vi "Software triggered acquisition - polling.vi"() -> ()   [LabVIEW 2015]
uses:
  SubVIs/Parameters Get & Set/Set Parameters/Set Gain.vi
  SubVIs/Parameters Get & Set/Get Parameters/Get NumberOfQueuedFrames.vi
  SubVIs/Parameters Get & Set/Set Parameters/Set ExposureTime_us.vi
  SubVIs/Parameters Get & Set/Set Parameters/Set FramesPerTrigger_zeroForUnlimited.vi
  SubVIs/Parameters Get & Set/Set Parameters/Set OperationMode.vi
  C:/code/Host/Installer/Scientific Camera Interfaces/LabVIEW/64_bit/Library_X64/Thorlabs.TSI.TLCameraInterfaces.dll
  64_bit/Library_X64/Thorlabs.TSI.TLCameraInterfaces.dll
panel:
  in  "Exposure (ms)":u32=100
  in  "Gain":u32 max=1023
  in  "Trigger Button":bool
  in  "stop":bool
  out "Intensity Graph Mono":u16[][](graph)
  out "FrameNumber":u32
  in  "Frames Per Trigger":u32=1
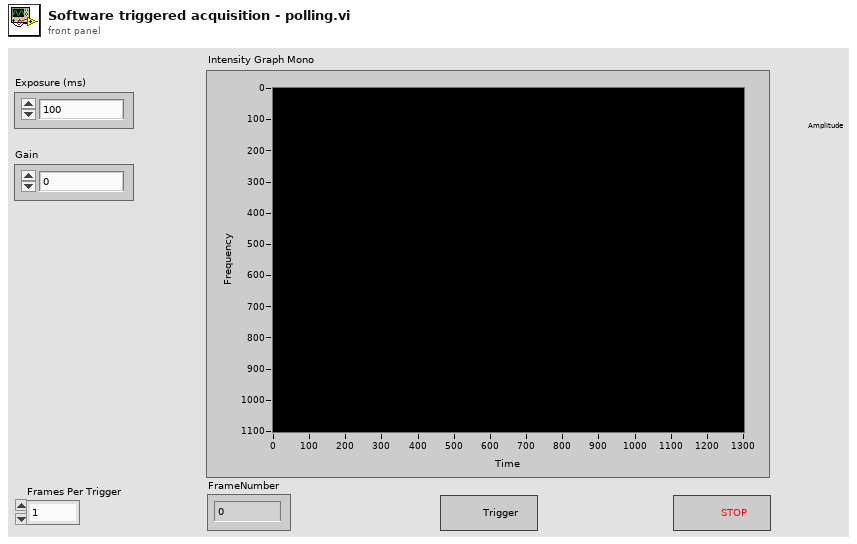
[diagram p1: front panel]
types:
  T1 = enum8{"Enabled", "Disabled", "Disabled and Grayed Out"}
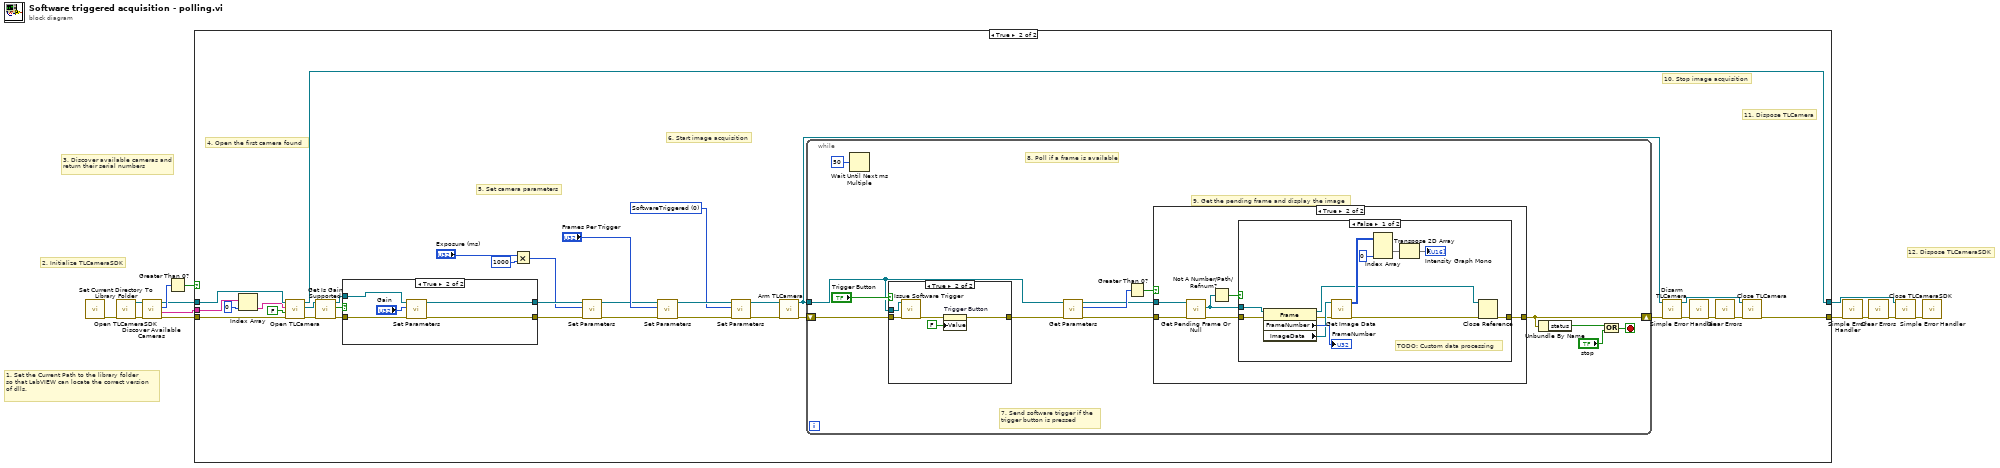
[diagram p0: block diagram]
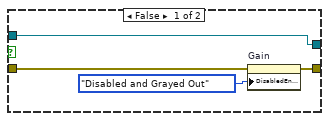
[diagram p3: hidden frame]
diagram:
  # "1. Set the Current Path to the library folder\nso that LabVIEW can locate the correct version\nof dlls."
  # "12. Dispose TLCameraSDK"
  # "3. Discover available cameras and\nreturn their serial numbers"
  # "2. Initialize TLCameraSDK"
  n1 = call "Set Current Directory To Library Folder.vi"() -> ("error out"=w7:errorcluster)  [unwired: 11 in]
  n2 = call "Open TLCameraSDK.vi"("error in (no error)"=w7) -> ("error out"=w6:errorcluster, "Thorlabs.TSI.TLCameraInterfaces.ITLCameraSDK"=w5:refnum<k24>)  [unwired: 9 in]
  n3 = call "Discover Available Cameras.vi"("error in (no error)"=w6, "Thorlabs.TSI.TLCameraInterfaces.ITLCameraSDK"=w5) -> ("error out"=w9:errorcluster, "Serial Numbers"=w11:string[], "Number of Cameras"=w13:i32, "Thorlabs.TSI.TLCameraInterfaces.ITLCameraSDK"=w10:refnum<k24>)  [unwired: 6 in]
  n4 = Greater Than 0?(x=w13) -> (x > 0?=w12:bool)
  n5 = case shown="True" w12 {
    tunnel: w11 -> [_ w48]
    tunnel: w10 -> [w14 w43]
    tunnel: w9 -> [w15 w32]
    tunnel: [w15 w30] -> w2
    tunnel: [w14 w42] -> w8
    frame False {
    }
    frame True {
      w18 = 0 items=["SoftwareTriggered", "HardwareTriggered", "Bulb", "Reserved1", "Reserved2"] ("OperationMode")
      # "11. Dispose TLCamera"
      # "10. Stop image acquisition"
      # "6. Start image acquisition"
      # "5. Set camera parameters"
      # "4. Open the first camera found"
      n6 = Index Array(array=w48, index=0) -> (element=w33:string)
      n7 = call "Open TLCamera.vi"("error in (no error)"=w32, "isDiagnosticsMessagesEnabled"=FALSE, "Camera serial number"=w33, "Thorlabs.TSI.TLCameraInterfaces.ITLCameraSDK"=w43) -> ("error out"=w35:errorcluster, "Thorlabs.TSI.TLCameraInterfaces.ITLCamera"=w34:refnum<k24>, "Thorlabs.TSI.TLCameraInterfaces.ITLCameraSDK"=w42:refnum<k24>)  [unwired: 5 in]
      n8 = call "Get Is Gain Supported.vi"("error in (no error)"=w35, "Thorlabs.TSI.TLCameraInterfaces.ITLCamera"=w34) -> ("error out"=w36:errorcluster, "Is Gain Supported?"=w38:bool, "Thorlabs.TSI.TLCameraInterfaces.ITLCamera"=w37:refnum<k24>)  [unwired: 7 in]
      n9 = case shown="True" w38 {
        tunnel: w37 -> [w50 w55]
        tunnel: w36 -> [w49 w57]
        tunnel: [w51 w56] -> w26
        tunnel: [w50 w54] -> w25
        frame False {
          n10 = property on="Gain" class="DigNum (strict)"(error in=w49, "DisabledEnum"=T1."Disabled and Grayed Out" ("Disabled")) -> (error out=w51:errorcluster)  [unwired: 1 in, 1 out]
        }
        frame True {
          n11 = call-poly "Set Parameters.vi"("error in (no error)"=w57, "Gain"="Gain", "Thorlabs.TSI.TLCameraInterfaces.ITLCamera"=w55) -> ("error out"=w56:errorcluster, "Thorlabs.TSI.TLCameraInterfaces.ITLCamera"=w54:refnum<k24>)  [unwired: 7 in]
        }
      }
      n12 = Multiply(x="Exposure (ms)", y=u32 1000) -> (x*y=w24:u32)
      n13 = call-poly "Set Parameters.vi"("error in (no error)"=w26, "ExposureTime_us"=w24, "Thorlabs.TSI.TLCameraInterfaces.ITLCamera"=w25) -> ("error out"=w22:errorcluster, "Thorlabs.TSI.TLCameraInterfaces.ITLCamera"=w21:refnum<k24>)  [unwired: 7 in]
      n14 = call-poly "Set Parameters.vi"("error in (no error)"=w22, "FramesPerTrigger_zeroForUnlimited"="Frames Per Trigger", "Thorlabs.TSI.TLCameraInterfaces.ITLCamera"=w21) -> ("error out"=w20:errorcluster, "Thorlabs.TSI.TLCameraInterfaces.ITLCamera"=w19:refnum<k24>)  [unwired: 7 in]
      n15 = call-poly "Set Parameters.vi"("error in (no error)"=w20, "OperationMode"=w18, "Thorlabs.TSI.TLCameraInterfaces.ITLCamera"=w19) -> ("error out"=w17:errorcluster, "Thorlabs.TSI.TLCameraInterfaces.ITLCamera"=w16:refnum<k24>)  [unwired: 7 in]
      n16 = call "Arm TLCamera.vi"("error in (no error)"=w17, "Thorlabs.TSI.TLCameraInterfaces.ITLCamera"=w16) -> ("error out"=w46:errorcluster, "Thorlabs.TSI.TLCameraInterfaces.ITLCamera"=w44:refnum<k24>)  [unwired: 8 in]
      n17 = while {
        tunnel: w44 -> [w61]
        shift-right: [w69] -> w31
        shift-left: w46 -> [w63]
        stop <- w66 stop-if-true
        # "7. Send software trigger if the \ntrigger button is pressed"
        # "9. Get the pending frame and display the image"
        # "8. Poll if a frame is available"
        n18 = Wait Until Next ms Multiple(millisecond multiple=u32 50) -> ()  [unwired: 1 out]
        n19 = case shown="True" "Trigger Button" {
          tunnel: w61 -> [_ w76]
          tunnel: w63 -> [w71 w73]
          tunnel: [w71 w74] -> w60
          frame False {
          }
          frame True {
            n20 = call "Issue Software Trigger.vi"("error in (no error)"=w73, "Thorlabs.TSI.TLCameraInterfaces.ITLCamera"=w76) -> ("error out"=w72:errorcluster)  [unwired: 8 in, 1 out]
            n21 = property on="Trigger Button" class="Bool (strict)"(error in=w72, "Value"=FALSE ("Trigger Button")) -> (error out=w74:errorcluster)  [unwired: 1 in, 1 out]
          }
        }
        n22 = call-poly "Get Parameters.vi"("error in (no error)"=w60, "Thorlabs.TSI.TLCameraInterfaces.ITLCamera"=w61) -> ("error out"=w59:errorcluster, "NumberOfQueuedFrames"=w62:i32, "Thorlabs.TSI.TLCameraInterfaces.ITLCamera"=w58:refnum<k24>)  [unwired: 7 in]
        n23 = Greater Than 0?(x=w62) -> (x > 0?=w70:bool)
        n24 = case shown="True" w70 {
          tunnel: w59 -> [w77 w80]
          tunnel: w58 -> [_ w83]
          tunnel: [w77 w81] -> w69
          frame False {
          }
          frame True {
            n25 = call "Get Pending Frame Or Null.vi"("error in (no error)"=w80, "Thorlabs.TSI.TLCameraInterfaces.ITLCamera"=w83) -> ("error out"=w78:errorcluster, "Thorlabs.TSI.TLCameraInterfaces.Frame"=w79:refnum<k24>)  [unwired: 7 in, 1 out]
            n26 = Not A Number/Path/Refnum?(number/path/refnum=w79) -> (NaN/Path/Refnum?=w82:bool)
            n27 = case shown="False" w82 {
              tunnel: w79 -> [w92 _]
              tunnel: w78 -> [w91 w96]
              tunnel: [w84 w96] -> w81
              frame False {
                # "TODO: Custom data processing"
                n28 = property class="Frame"(reference=w92, error in=w91) -> (reference out=w85:refnum<k24>, error out=w87:errorcluster, "FrameNumber"=→"FrameNumber":u32, "ImageData"=w89:refnum<k24>)
                n29 = call "Get Image Data.vi"("error in (no error)"=w87, "Thorlabs.TSI.ImageDataInterfaces.IImageData"=w89) -> ("error out"=w86:errorcluster, "Frame Data"=w88:u16[][][])  [unwired: 6 in, 2 out]
                n30 = Index Array(array=w88, index (dim 2)=0 ("disabled index (col)")) -> (element=w93:u16[][])  [unwired: 2 in]
                n31 = Transpose 2D Array(2D array=w93) -> (transposed array=→"Intensity Graph Mono":u16[][])
                n32 = Close Reference(reference=w85, error in (no error)=w86) -> (error out=w84:errorcluster)
              }
              frame True {
              }
            }
          }
        }
        n33 = Unbundle By Name(w69) -> ("status"=w68:bool)
        n34 = Or(x=w68, y="stop") -> (x .or. y?=w66:bool)
      }
      n35 = call "Disarm TLCamera.vi"("error in (no error)"=w31, "Thorlabs.TSI.TLCameraInterfaces.ITLCamera"=w44) -> ("error out"=w29:errorcluster, "Thorlabs.TSI.TLCameraInterfaces.ITLCamera"=w45:refnum<k24>)  [unwired: 8 in]
      n36 = call <vilib>:"Simple Error Handler.vi"("error in (no error)"=w29) -> ("error out"=w28:errorcluster)  [unwired: 4 in, 4 out]
      n37 = call <vilib>:"Clear Errors.vi"("error in (no error)"=w28) -> ("error out"=w27:errorcluster)  [unwired: 5 in, 1 out]
      n38 = call "Close TLCamera.vi"("error in (no error)"=w27, "Thorlabs.TSI.TLCameraInterfaces.ITLCamera"=w45) -> ("error out"=w30:errorcluster)  [unwired: 9 in]
    }
  }
  n39 = call <vilib>:"Simple Error Handler.vi"("error in (no error)"=w2) -> ("error out"=w3:errorcluster)  [unwired: 4 in, 4 out]
  n40 = call <vilib>:"Clear Errors.vi"("error in (no error)"=w3) -> ("error out"=w1:errorcluster)  [unwired: 5 in, 1 out]
  n41 = call "Close TLCameraSDK.vi"("error in (no error)"=w1, "Thorlabs.TSI.TLCameraInterfaces.ITLCameraSDK"=w8) -> ("error out"=w4:errorcluster)  [unwired: 9 in]
  n42 = call <vilib>:"Simple Error Handler.vi"("error in (no error)"=w4) -> ()  [unwired: 4 in, 5 out]
